vi "Initialize.vi"(6 "Start Direction":T1=enum."E", 8 "error in (no error)":errorcluster, 9 "Kamikaze DVR":T2, 10 "SquareStatus DVR":T3, 11 "Mother in":refnum<class "Formics.lvclass">) -> (0 "error out":errorcluster, 3 "Mother out":refnum<class "Formics.lvclass">)   [LabVIEW 2015, in "Formics.lvclass"]
uses:
  Formics.lvclass
  SquareStatus DVR.ctl
  Kamikaze DVR.ctl
  Type Defs/Direction Enum.ctl
  Action Queue Element.ctl
  Type Defs/Action Enum.ctl
  Formics.lvclass/Formics.ctl
  Type Defs/SB Type Defs.lvlib
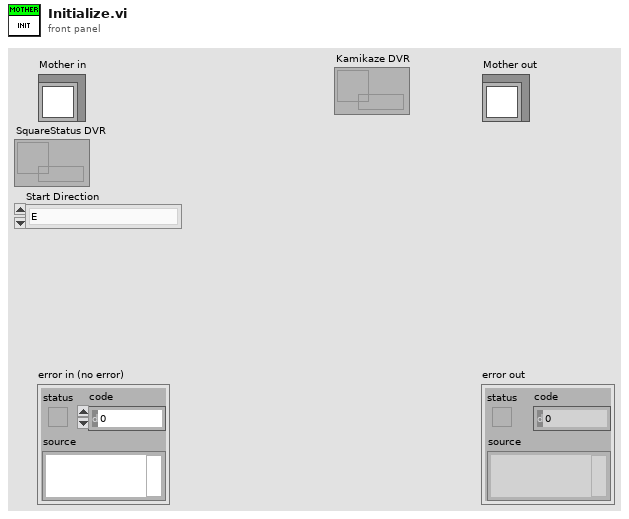
[diagram p1: front panel]
types:
  T1 = typedef "SB Type Defs.lvlib/Direction Enum.ctl" = enum16{"NW", "N", "NE", "E", "SE", "S", "SW", "W"}
  T2 = typedef "Formics.lvclass/Kamikaze DVR.ctl" = refnum<data-value>
  T3 = typedef "Formics.lvclass/SquareStatus DVR.ctl" = refnum<data-value>
  T4 = typedef "Formics.lvclass/Action Queue Element.ctl" = cluster{"Action":T5, "Times":i32}
  T5 = typedef "SB Type Defs.lvlib/Action Enum.ctl" = enum16{"Wait", "Move", "Attack", "Replicate"}
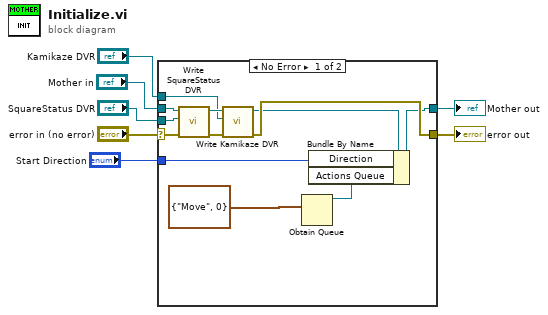
[diagram p0: block diagram]
diagram:
  n1 = case shown="No Error" "error in (no error)" {
    selector: "error in (no error)" -> [w19 w21]
    tunnel: [w13 w21] -> w6
    tunnel: [w11 w20] -> w4
    tunnel: "Mother in" -> [w17 w20]
    tunnel: "SquareStatus DVR" -> [w16 _]
    tunnel: "Kamikaze DVR" -> [w14 _]
    tunnel: "Start Direction" -> [w10 _]
    frame No Error {
      n2 = call-dynamic "Write SquareStatus DVR.vi"("error in (no error)"=w19, "data value reference"=w16, "Mother in"=w17) -> ("error out"=w18:errorcluster, "Mother out"=w15:refnum<class "Formics.lvclass">)  [unwired: 7 in]
      n3 = call "Write Kamikaze DVR.vi"("error in (no error)"=w18, "Kamikaze DVR"=w14, "Mother in"=w15) -> ("error out"=w13:errorcluster, "Mother out"=w12:refnum<class "Formics.lvclass">)  [unwired: 7 in]
      n4 = Obtain Queue(element data type=T4 {"Action"=enum."Move", "Times"=0}) -> (queue out=w8:refnum<queue>)  [unwired: 4 in, 2 out]
      n5 = Bundle By Name(cluster=w12, "Direction"=w10, "Actions Queue"=w8) -> (w11:refnum<class "Formics.lvclass">)
    }
    frame Error {
    }
  }
  "error out" <- w6
  "Mother out" <- w4
